vi "Motor_Speed_Computation.vi"(8 "Contracted muscle":T1(ring)=enum."Triceps contracted", 9 "Motor type":enum16{"Mover4 motors", "Dynamixel motors"}(ring), 10 "EMG signal max amplitude (V)":dbl, 11 "EMG signal mean amplitude (V)":dbl) -> (2 "Motor speed (RPM or bit)":dbl)   [LabVIEW 2015]
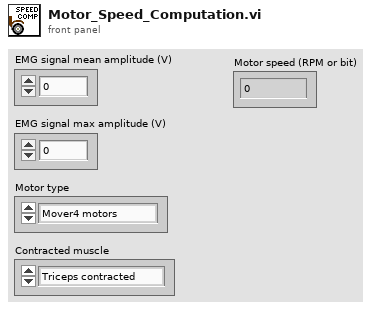
[diagram p1: front panel]
types:
  T1 = enum16{"Biceps contracted", "Triceps contracted"}
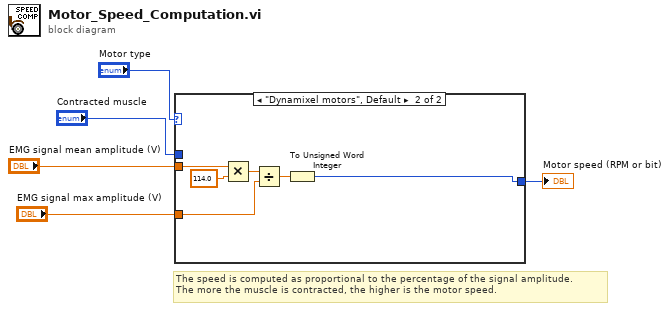
[diagram p0: block diagram]
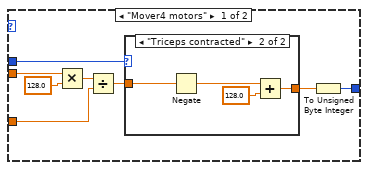
[diagram p2: hidden frame]
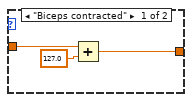
[diagram p3: hidden frame]
diagram:
  # "The speed is computed as proportional to the percentage of the signal amplitude.\nThe more the muscle is contracted, the higher is the motor speed."
  n1 = case shown="\"Dynamixel motors\", Default" "Motor type" {
    tunnel: "EMG signal mean amplitude (V)" -> [w12 w26]
    tunnel: "EMG signal max amplitude (V)" -> [w9 w23]
    tunnel: [w6 w21] -> w2
    tunnel: "Contracted muscle" -> [w13 _]
    frame "Mover4 motors" {
      n2 = Multiply(x=w12, y=128.0) -> (x*y=w10:dbl)
      n3 = Divide(x=w10, y=w9) -> (x/y=w8:dbl)
      n4 = case shown="\"Triceps contracted\"" w13 {
        tunnel: w8 -> [w16 w20]
        tunnel: [w14 w18] -> w7
        frame "Biceps contracted" {
          n5 = Add(x=w16, y=127.0) -> (x+y=w14:dbl)
        }
        frame "Triceps contracted" {
          n6 = Negate(x=w20) -> (-x=w19:dbl)
          n7 = Add(x=w19, y=128.0) -> (x+y=w18:dbl)
        }
      }
      n8 = To Unsigned Byte Integer(number=w7) -> (unsigned 8bit integer=w6:u8)
    }
    frame "Dynamixel motors", Default {
      n9 = Multiply(x=w26, y=114.0) -> (x*y=w24:dbl)
      n10 = Divide(x=w24, y=w23) -> (x/y=w22:dbl)
      n11 = To Unsigned Word Integer(number=w22) -> (unsigned 16bit integer=w21:u16)
    }
  }
  "Motor speed (RPM or bit)" <- w2
